vi "while.vi"() -> ()   [LabVIEW 2020]
panel:
  out "Array":i32[](array[numeric])
  out "Numeric 2":i32
  in  "Knob":dbl(knob) scale=0.0..100.0
  out "Thermometer":dbl(slide) scale=0.0..100.0
  out "Numeric":i32
  in  "stop":bool
  # "while"
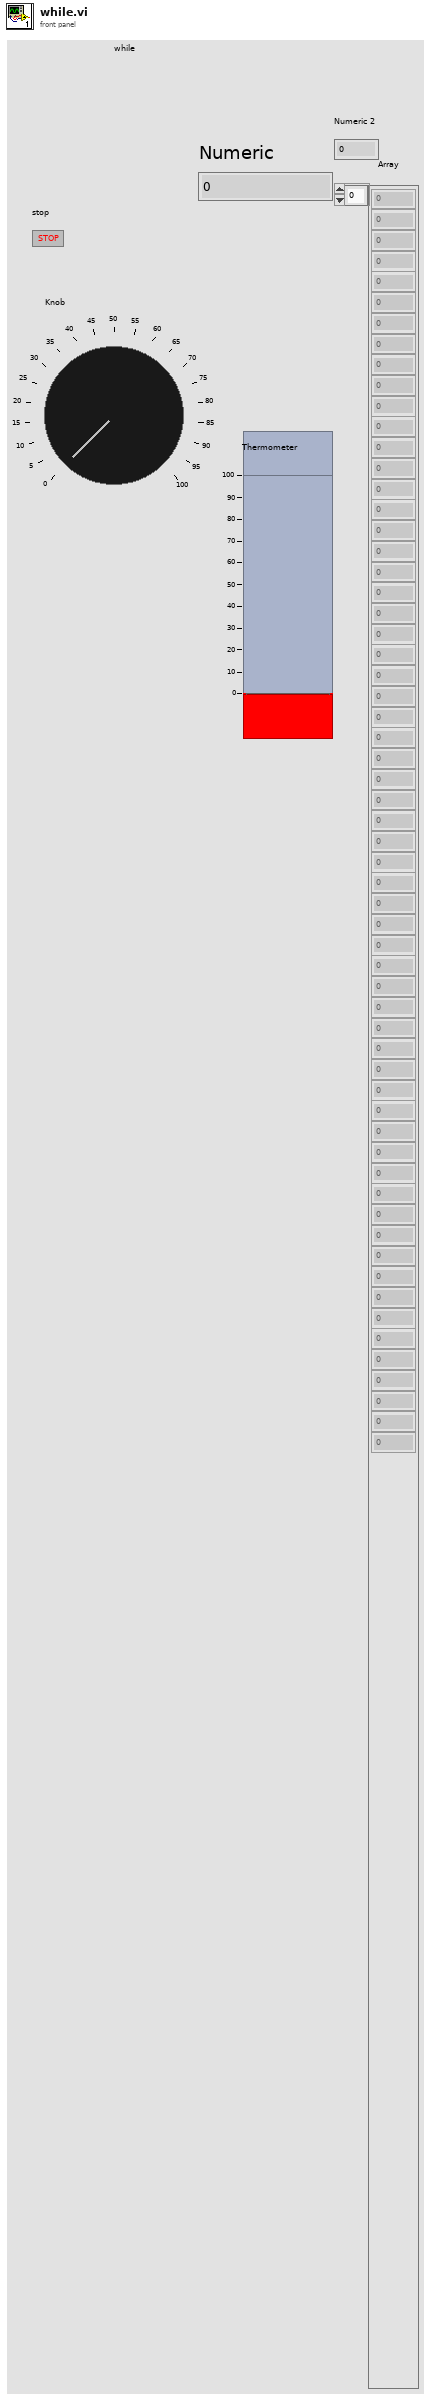
[diagram p1: front panel]
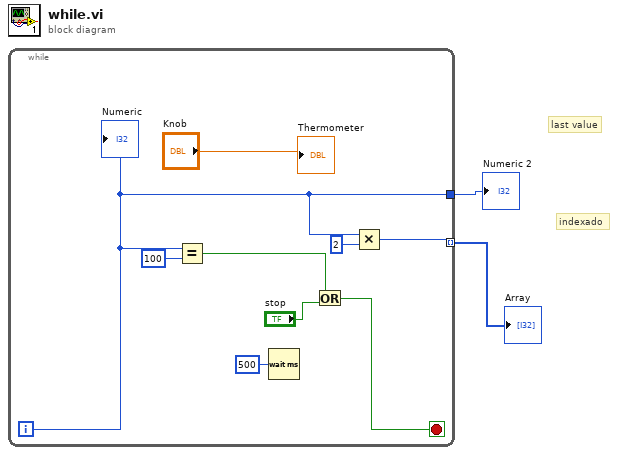
[diagram p0: block diagram]
diagram:
  # "indexado"
  # "last value"
  n1 = while {
    tunnel: [w5] -> w2
    tunnel: [w3] -> w1 mode=indexing
    i -> [w5]
    stop <- w6 stop-if-true
    n2 = Equal?(x=w5, y=100) -> (x = y?=w7:bool)
    n3 = Wait (ms)(milliseconds to wait=u32 500) -> ()  [unwired: 1 out]
    n4 = Or(x=w7, y="stop") -> (x .or. y?=w6:bool)
    n5 = Multiply(x=w5, y=2) -> (x*y=w3:i32)
    "Numeric" <- w5
    "Thermometer" <- "Knob"
  }
  "Numeric 2" <- w2
  "Array" <- w1
